vi "ActiveObjects_DynamicEvents_SendMsgToProcess_5x6x5_Singleton.vi"(5 "DataToProcess":variant, 11 "Error In":errorcluster) -> (15 "Error Out":errorcluster)   [LabVIEW 2020]
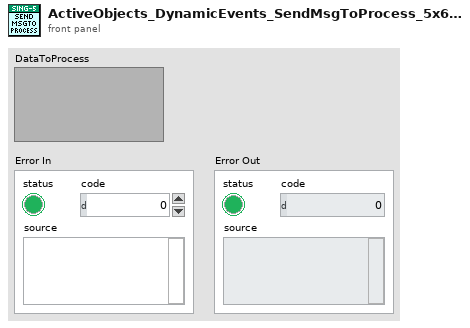
[diagram p1: front panel]
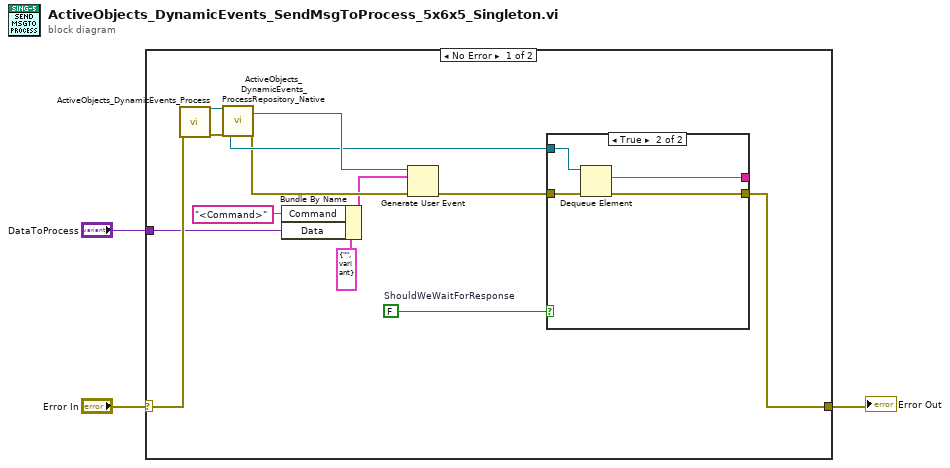
[diagram p0: block diagram]
diagram:
  n1 = case shown="No Error" "Error In" {
    selector: "Error In" -> [w9 w22]
    tunnel: [w11 w22] -> w2
    tunnel: "DataToProcess" -> [w5 _]
    frame No Error {
      w15 = FALSE  # ShouldWeWaitForResponse
      n2 = call <resource>:"ActiveObjects_DynamicEvents_Process.vi"("error in"=w9) -> ("reference out"=w10:refnum<class>, "error out"=w8:errorcluster)  [unwired: 17 in]
      n3 = call <resource>:"ActiveObjects_DynamicEvents_ProcessRepository_Native.vi"("reference in"=w10, "Error In"=w8) -> ("QueueFromProcess"=w13:refnum<queue>, "EventsToProcess"=w16:refnum<user-event>, "Error Out"=w12:errorcluster)  [unwired: 10 in, 5 out]
      n4 = Bundle By Name(cluster=cluster{"Command":string, "Data":variant} {"Command"="", "Data"=variant} ("MessageToProcess"), "Command"="<Command>", "Data"=w5) -> (w6:cluster{"Command":string, "Data":variant})
      n5 = Generate User Event(user event=w16, event data cluster=w6, error in=w12) -> (error out=w14:errorcluster)  [unwired: 1 in, 1 out]
      n6 = case shown="True" w15 {
        tunnel: w14 -> [w17 w21]
        tunnel: w13 -> [_ w20]
        tunnel: [_ w19] -> _
        tunnel: [w17 w18] -> w11
        frame False {
        }
        frame True {
          n7 = Dequeue Element(queue=w20, error in (no error)=w21) -> (element=w19:string, error out=w18:errorcluster)  [unwired: 1 in, 2 out]
        }
      }
    }
    frame Error {
    }
  }
  "Error Out" <- w2
